vi "filterRobotVelocityPeak.vi"(5 "last_robots":T1[](array[typedef]) {"height" format="%+4.3f"; "pixel_y" format="%+4.3f"; "pixel_x" format="%+4.3f"; "orientation" format="%+4.3f"; "y" format="%+4.3f"; "confidence" format="%4.3f"; "x" format="%+4.3f"}, 7 "dt":dbl, 8 "robot_id":u32, 9 "vel_y":dbl, 10 "vel_x":dbl, 11 "Vision in":refnum<class "Vision.lvclass">) -> (1 "vel_y out":dbl, 2 "vel_x out":dbl, 3 "Vision out":refnum<class "Vision.lvclass">)   [LabVIEW 2023, in "Vision.lvclass"]
uses:
  Vision.lvclass
  Old vision/Controls/SSL Detection Robot.ctl
  <vilib>/Analysis/Matrix/Datatypes/RealMatrix.ctl
  <vilib>/Analysis/Matrix/NI_Matrix.lvlib
panel:
  out "error out":errorcluster
  in  "error in (no error)":errorcluster
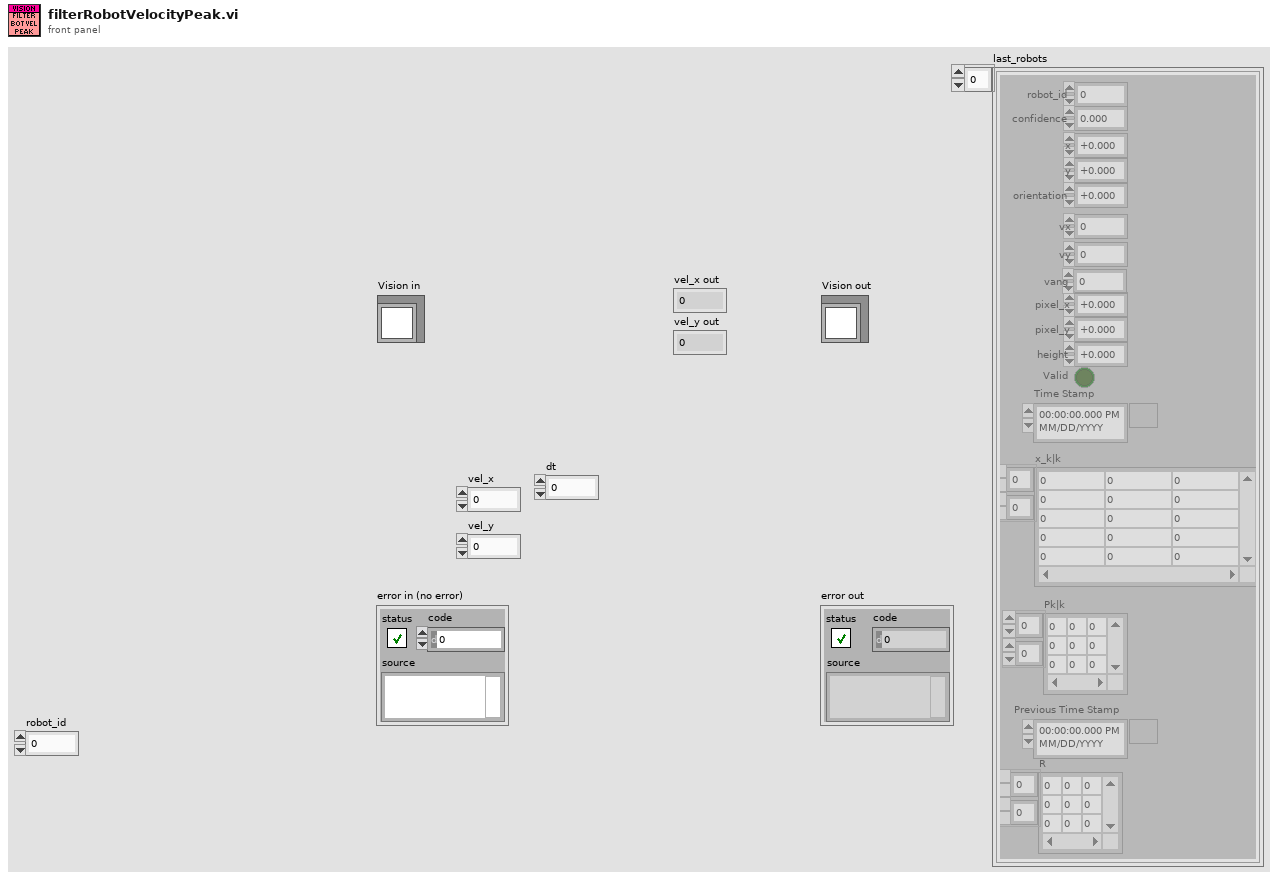
[diagram p1: front panel]
types:
  T1 = typedef "SSL Detection Robot.ctl" = cluster{"x":sgl, "robot_id":u32, "confidence":sgl, "y":sgl, "orientation":sgl, "pixel_x":sgl, "pixel_y":sgl, "height":sgl, "Valid":bool, "Time Stamp":timestamp, "x_k|k":T2, "Pk|k":T2, "Previous Time Stamp":timestamp, "R":T2, "vx":dbl, "vy":dbl, "vang":dbl}
  T2 = typedef "NI_Matrix.lvlib/RealMatrix.ctl" = dbl[][]
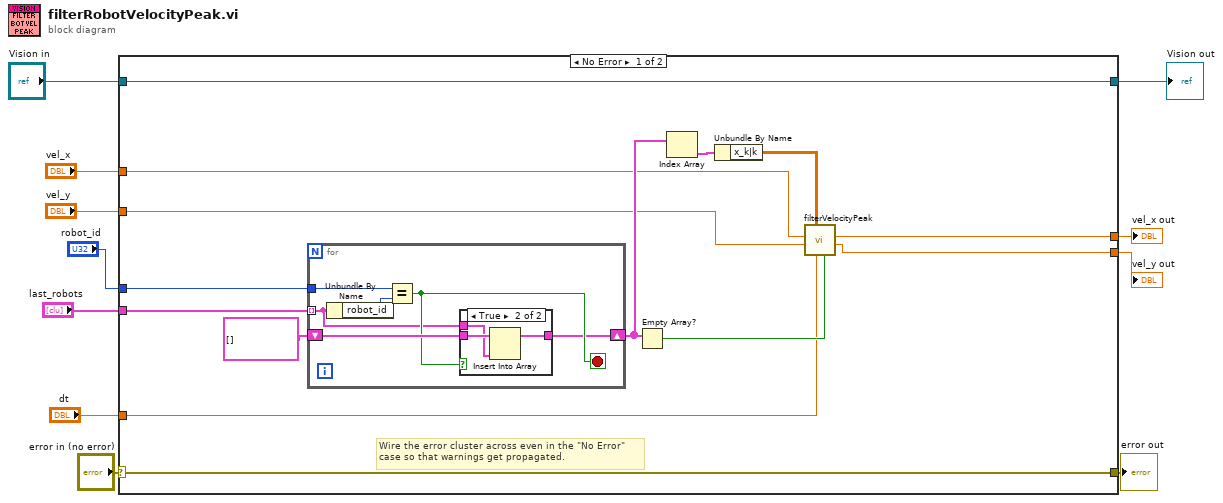
[diagram p0: block diagram]
diagram:
  n1 = case shown="No Error" "error in (no error)" {
    selector: "error in (no error)" -> [w24 w37]
    tunnel: [w24 w37] -> w10
    tunnel: [w25 w36] -> w8
    tunnel: "Vision in" -> [w25 w36]
    tunnel: "robot_id" -> [w23 _]
    tunnel: "vel_x" -> [w18 _]
    tunnel: "dt" -> [w17 _]
    tunnel: "vel_y" -> [w16 _]
    tunnel: [w15 _] -> w3
    tunnel: [w14 _] -> w2
    tunnel: "last_robots" -> [w13 _]
    frame No Error {
      # "Wire the error cluster across even in the \"No Error\"\ncase so that warnings get propagated."
      n2 = for {
        tunnel: w23 -> [w31]
        shift-right: [w27] -> w22
        shift-left: T1[] [] -> [w29]
        tunnel: w13 -> [w26] mode=indexing
        stop <- w28 stop-if-true
        n3 = Unbundle By Name(w26) -> ("robot_id"=w30:u32)
        n4 = Equal?(x=w31, y=w30) -> (x = y?=w28:bool)
        n5 = case shown="True" w28 {
          tunnel: w29 -> [w32 w35]
          tunnel: [w32 w34] -> w27
          tunnel: w26 -> [_ w33]
          frame False {
          }
          frame True {
            n6 = Insert Into Array(array=w35, new element=w33) -> (w34:T1[])  [unwired: 1 in]
          }
        }
      }
      n7 = Empty Array?(array=w22) -> (empty?=w19:bool)
      n8 = Index Array(array=w22) -> (element=w21:T1)  [unwired: 1 in]
      n9 = Unbundle By Name(w21) -> ("x_k|k"=w20:T2)
      n10 = call "filterVelocityPeak.vi"("empty?"=w19, "dt"=w17, "x_k|k"=w20, "vel_y"=w16, "vel_x"=w18) -> ("vel_y out"=w14:dbl, "vel_x out"=w15:dbl)  [unwired: 3 in, 2 out]
    }
    frame Error {
    }
  }
  "error out" <- w10
  "Vision out" <- w8
  "vel_x out" <- w3
  "vel_y out" <- w2
